vi "deadzone.vi"(8 "min":dbl, 9 "max":dbl, 10 "x":dbl) -> (2 "dead zone":dbl)   [LabVIEW 2015]
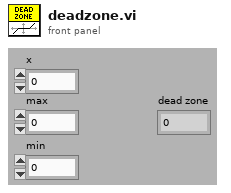
[diagram p1: front panel]
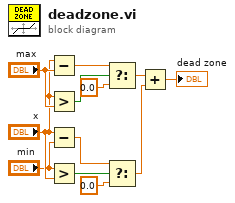
[diagram p0: block diagram]
diagram:
  n1 = Subtract(x="x", y="max") -> (x-y=w10:dbl)
  n2 = Greater?(x="x", y="max") -> (0:w12:bool)
  n3 = Subtract(x="x", y="min") -> (x-y=w5:dbl)
  n4 = Greater?(x="min", y="x") -> (0:w6:bool)
  n5 = Select(t=w10, s=w12, f=0.0) -> (s? t:f=w2:dbl)
  n6 = Select(t=w5, s=w6, f=0.0) -> (s? t:f=w1:dbl)
  n7 = Add(x=w2, y=w1) -> (x+y=→"dead zone":dbl)
